vi "Configure Gamepad.vi"(4 "invert z":refnum<vi>, 6 "Cluster":T3, 7 "Configuration":T2, 8 "Slide 2":refnum<vi>, 9 "invert y":refnum<vi>, 10 "invert x":refnum<vi>, 11 "device ID":refnum<k1>) -> (3 "Configuration":T2)   [LabVIEW 2012]
uses:
  <vilib>/Utility/miscctls.llb/LVPointTypeDef.ctl
  <vilib>/Utility/inputDevices.llb/joystickAcquire.vi
  <vilib>/Utility/file.llb/Write To Spreadsheet File (I64).vi
  <vilib>/Utility/file.llb/Read From Spreadsheet File (I64).vi
panel:
  in  "Invert":bool=TRUE
  out "Settings Refrences":T1
  in  "M3+":u16(ring)=8 items=["1 X"=1, "2 A"=2, "3 B"=3, "4 Y"=4, "5 LB"=5, "6 RB"=6, "7 LT"=7, "8 RT"=8, "9 Back"=9]
  in  "M3-":u16(ring)=6 items=["1 X"=1, "2 A"=2, "3 B"=3, "4 Y"=4, "5 LB"=5, "6 RB"=6, "7 LT"=7, "8 RT"=8, "9 Back"=9]
  out "down":u16(ring) items=["M1+", "M1-", "M2+", "M2-"]
  out "left":u16(ring) items=["M1+", "M1-", "M2+", "M2-"]
  in  "right":u16(ring) items=["M1+", "M1-", "M2+", "M2-"]
  out "V":i32
  out "U":i32
  out "Left Y":i32
  out "B":i32
  out "A":i32
  out "Left X":i32
  out "Right Y":i32
  out "Right X":i32
  in  "close_button":bool
  in  "up":u16(ring) items=["M1+", "M1-", "M2+", "M2-"]
  in  "load":bool
  in  "save":bool
  in  "Invert":bool
  in  "Invert":bool=TRUE
  in  "Slide":cluster{u32, u32, u32}(slide)={7, 6, 2} scale=0.0..7.0
  in  "xr":u16(ring)=1 items=["1 X"=1, "2 A"=2, "3 B"=3, "4 Y"=4, "5 LB"=5, "6 RB"=6, "7 LT"=7, "8 RT"=8, "9 Back"=9]
  in  "yf":u16(ring)=4 items=["1 X"=1, "2 A"=2, "3 B"=3, "4 Y"=4, "5 LB"=5, "6 RB"=6, "7 LT"=7, "8 RT"=8, "9 Back"=9]
  in  "yr":u16(ring)=2 items=["1 X"=1, "2 A"=2, "3 B"=3, "4 Y"=4, "5 LB"=5, "6 RB"=6, "7 LT"=7, "8 RT"=8, "9 Back"=9]
  in  "xf":u16(ring)=3 items=["1 X"=1, "2 A"=2, "3 B"=3, "4 Y"=4, "5 LB"=5, "6 RB"=6, "7 LT"=7, "8 RT"=8, "9 Back"=9]
  in  "halt 2":u16(ring)=9 items=["1 X"=1, "2 A"=2, "3 B"=3, "4 Y"=4, "5 LB"=5, "6 RB"=6, "7 LT"=7, "8 RT"=8, "9 Back"=9]
  # "Control-sticks"
  # "Button mapping"
  # "Instructions\nDrag the M1 (green), M2 (red), and M3 (Blue)  MicroDrive-axis selectors to the name of a Gamepad Control-stick. \nNOTE: To identify your desired Control-stick, toggle the Control-stick while watching \"Readings\".\n\n."
  # "Instructions:\nClick on the text in a square to list Gamepad button options. The selected button will move the corresponding axis of the MicroDrive.\n\nThese settings effect the Gamepad buttons, and the  buttons/limit-lights of the main window."
  # "Axis"
  # "Selection"
  # "Readings"
  # "M1 Axis"
  # "M2 Axis"
  # "M3 Axis"
  # "CAUTION: The Gamepad's \"Mode\" button will disable the Control-sticks"
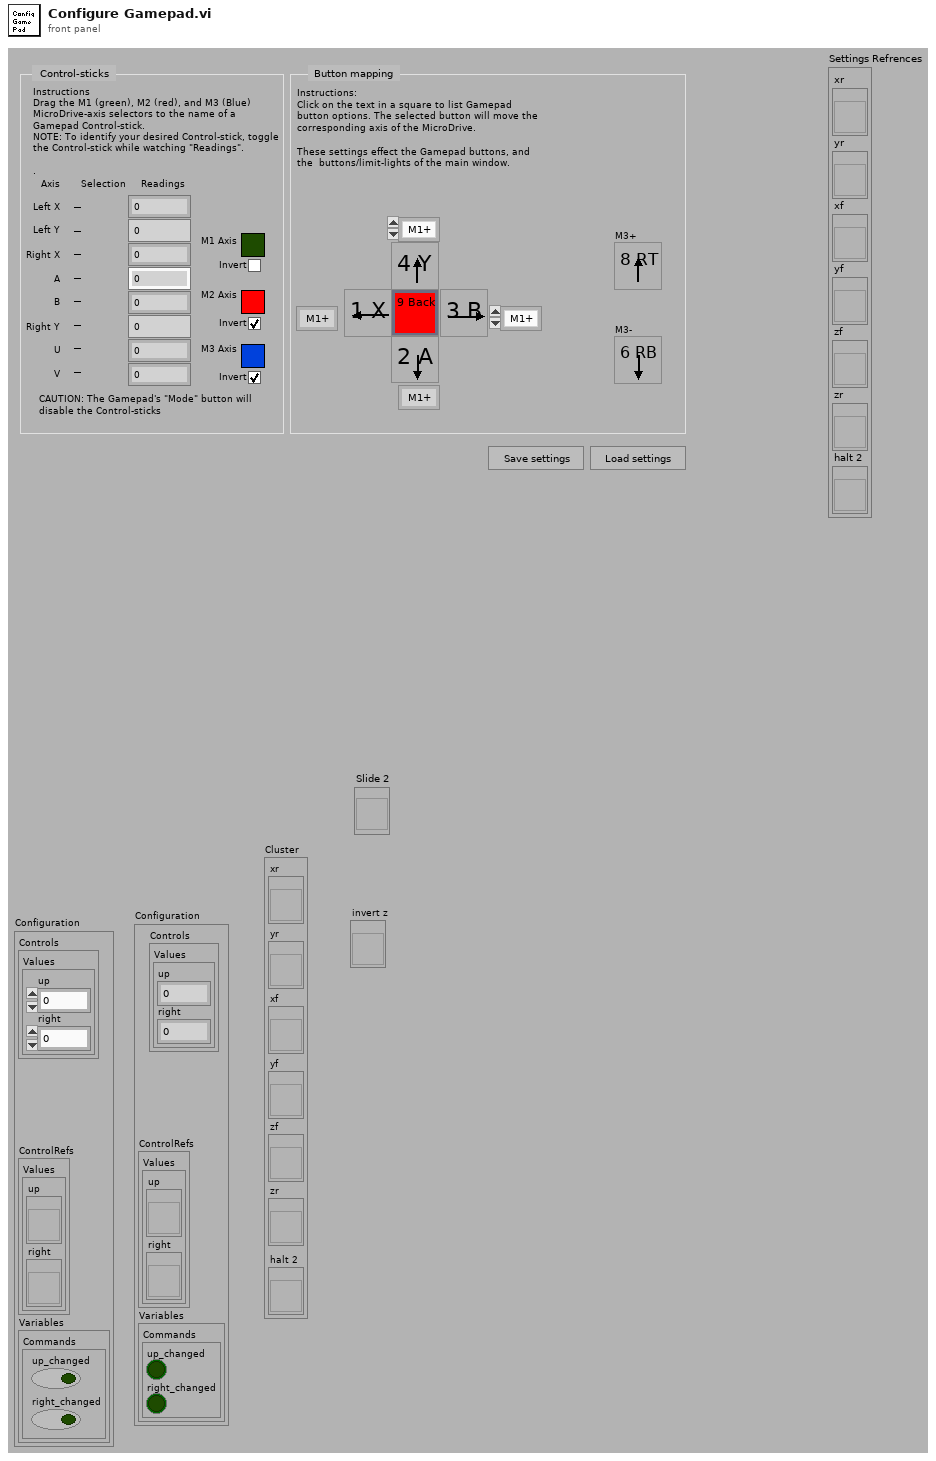
[diagram p1: front panel]
types:
  T1 = cluster{"xr":refnum<vi>, "yr":refnum<vi>, "xf":refnum<vi>, "yf":refnum<vi>, "zf":refnum<vi>, "zr":refnum<vi>, "halt 2":refnum<vi>}
  T2 = cluster{"Controls":cluster{"Values":cluster{"up":u16, "right":u16}}, "ControlRefs":cluster{"Values":cluster{"up":refnum<vi>, "right":refnum<vi>}}, "Variables":cluster{"Commands":cluster{"up_changed":bool, "right_changed":bool}}}
  T3 = cluster{"xr":refnum<vi>, "yr":refnum<vi>, "xf":refnum<vi>, "yf":refnum<vi>, "zr":refnum<vi>, "zf":refnum<vi>, "halt 2":refnum<vi>}
  T4 = typedef "LVPointTypeDef.ctl" = cluster{"Horizontal":i16, "Vertical":i16}
  T5 = cluster{"xr":refnum<vi>, "yr":refnum<vi>, "xf":refnum<vi>, "yf":refnum<vi>, "M3+":refnum<vi>, "M3-":refnum<vi>, "halt 2":refnum<vi>}
  T6 = cluster{"X axis":i32, "Y axis":i32, "Z axis":i32, "X axis rotation":i32, "Y axis rotation":i32, "Z axis rotation":i32, "U axis":i32, "V axis":i32}
  T7 = cluster{"Right X axis":i32, "Right Y axis":i32, "Left X axis":i32, "A Axis":i32, "B Axis":i32, "Left Y axis":i32, "U axis":i32, "V axis":i32}
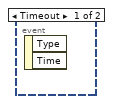
[diagram p2: hidden frame]
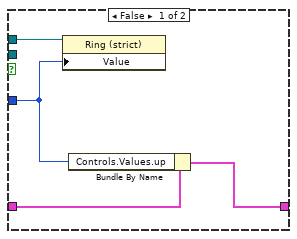
[diagram p4: hidden frame]
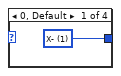
[diagram p5: hidden frame]
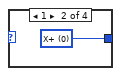
[diagram p6: hidden frame]
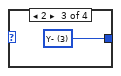
[diagram p7: hidden frame]
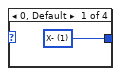
[diagram p8: hidden frame]
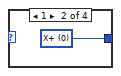
[diagram p9: hidden frame]
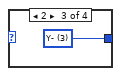
[diagram p10: hidden frame]
diagram:
  n1 = flat-sequence {
    tunnel: ["Configuration"] -> w9
    tunnel: w9 -> [w27]
    tunnel: [w26] -> w8
    tunnel: w8 -> [w29]
    tunnel: [w29] -> w22
    tunnel: [w28] -> w21
    tunnel: w22 -> [w31]
    tunnel: [w31] -> w20
    tunnel: w21 -> [w30]
    tunnel: [w35] -> w19
    tunnel: [w34] -> w18
    tunnel: w20 -> [w34]
    tunnel: [w44] -> w17
    tunnel: w19 -> [w44]
    tunnel: w18 -> [w43]
    tunnel: [w43] -> w16
    tunnel: w17 -> [w71]
    tunnel: [w71] -> w4
    tunnel: [w55] -> w2
    tunnel: w16 -> [w55]
    tunnel: w4 -> [w80]
    tunnel: [w80] -> w3
    tunnel: w2 -> [w79]
    tunnel: [w79] -> w1
    tunnel: [w82] -> w15
    tunnel: w3 -> [w82]
    tunnel: [w81] -> w14
    tunnel: w1 -> [w81]
    tunnel: w15 -> [w84]
    tunnel: [w84] -> w13
    tunnel: w14 -> [w83]
    tunnel: [w83] -> w12
    tunnel: w13 -> [w90]
    tunnel: w12 -> [w86]
    tunnel: [w88] -> w11
    tunnel: [w87] -> w10
    tunnel: w11 -> [w359]
    tunnel: w10 -> [w358]
    tunnel: [w359] -> w7
    tunnel: [w358] -> w5
    tunnel: w7 -> [w362]
    tunnel: [w362] -> w6
    tunnel: w5 -> [w361]
    tunnel: w6 -> [w363]
    frame #0 {
    }
    frame #1 {
      n2 = control-ref of="up"() -> (w25:refnum<vi>)
      n3 = control-ref of="right"() -> (w24:refnum<vi>)
      n4 = Bundle By Name(cluster=w27, "ControlRefs.Values.up"=w25, "ControlRefs.Values.right"=w24) -> (w26:T2)
    }
    frame #2 {
      n5 = control-ref of="This VI"() -> (w28:refnum<vi>)
    }
    frame #3 {
      w32 = FALSE ("Front Panel Window:Show Menu Bar")
      n6 = property class="VI"(reference=w30, "Front Panel.Minimizeable"=w32) -> ()  [unwired: 1 in, 2 out]
      n7 = property class="VI"(reference=w30, "Front Panel.ShowMenuBar"=w32) -> ()  [unwired: 1 in, 2 out]
      n8 = property class="VI"(reference=w30, "TB.Visible"=w32) -> ()  [unwired: 1 in, 2 out]
      n9 = property class="VI"(reference=w30, "Front Panel.Resizeable"=w32) -> ()  [unwired: 1 in, 2 out]
      n10 = property class="VI"(reference=w30, "Front Panel.Title"="Configure Gamepad" ("Front Panel Window:Title")) -> ()  [unwired: 1 in, 2 out]
    }
    frame #4 {
      n11 = control-ref of="This VI"() -> (w35:refnum<vi>)
      n12 = control-ref of="Pane"() -> (w36:refnum<vi>)
      n13 = property class="Pane"(reference=w36, "Origin"=T4 {"Horizontal"=0, "Vertical"=0}) -> ()  [unwired: 1 in, 2 out]
      n14 = property class="VI"(reference=w35, "GrowByDefault"=TRUE ("Expand When Dropped As SubVI")) -> ()  [unwired: 1 in, 2 out]
    }
    frame #5 {
      n15 = control-ref of="M3+"() -> (w39:refnum<vi>)
      n16 = control-ref of="halt 2"() -> (w42:refnum<vi>)
      n17 = control-ref of="M3-"() -> (w40:refnum<vi>)
      n18 = control-ref of="xr"() -> (w48:refnum<vi>)
      n19 = control-ref of="yr"() -> (w47:refnum<vi>)
      n20 = control-ref of="xf"() -> (w46:refnum<vi>)
      n21 = control-ref of="yf"() -> (w45:refnum<vi>)
      n22 = Bundle("xr"=w48, "yr"=w47, "xf"=w46, "yf"=w45, "M3+"=w39, "M3-"=w40, "halt 2"=w42) -> (→"Settings Refrences":T5)  [unwired: 1 out]
    }
    frame #6 {
      w50 = u32 7 ("x")
      n23 = local read "Settings Refrences"() -> (w54:T1)
      n24 = local read "Slide 2"() -> (w53:refnum<vi>)
      n25 = local read "Cluster"() -> (w58:T3)
      n26 = local read "invert x"() -> (w57:refnum<vi>)
      n27 = local read "invert y"() -> (w56:refnum<vi>)
      n28 = property on="Property Node" class="Slide (strict)"(reference=w53) -> ("Value"=w66:cluster{u32, u32, u32})  [unwired: 1 in, 2 out]
      n29 = Cluster To Array(cluster=w58) -> (array=w69:refnum<vi>[])
      n30 = Cluster To Array(cluster=w54) -> (array=w70:refnum<vi>[])
      n31 = property on="Property Node" class="Bool (strict)"(reference=w56) -> ("Value"=w62:bool)  [unwired: 1 in, 2 out]
      n32 = property on="Property Node" class="Bool (strict)"(reference=w57) -> ("Value"=w68:bool)  [unwired: 1 in, 2 out]
      n33 = for {
        tunnel: w70 -> [w73] mode=indexing
        tunnel: w69 -> [w74] mode=indexing
        n34 = property on="Property Node" class="Ring (strict)"(reference=w74) -> ("Value"=w72:u16)  [unwired: 1 in, 2 out]
        n35 = property on="Property Node" class="Ring (strict)"(reference=w73, "Value"=w72) -> ()  [unwired: 1 in, 2 out]
      }
      n36 = control-ref of="invert y"() -> (w59:refnum<vi>)
      n37 = Unbundle(w66) -> (w65:u32, w64:u32, w49:u32)
      n38 = control-ref of="invert x"() -> (w61:refnum<vi>)
      n39 = Subtract(x=w50, y=w65) -> (x-y=w52:u32)
      n40 = Subtract(x=w50, y=w64) -> (x-y=w63:u32)
      n41 = Subtract(x=w50, y=w49) -> (x-y=w51:u32)
      n42 = property on="Property Node" class="Bool (strict)"(reference=w59, "Value"=w62) -> ()  [unwired: 1 in, 2 out]
      n43 = property on="Property Node" class="Bool (strict)"(reference=w61, "Value"=w68) -> ()  [unwired: 1 in, 2 out]
      n44 = control-ref of="Slide"() -> (w60:refnum<vi>)
      n45 = Bundle(w52, w63, w51) -> (w67:cluster{u32, u32, u32})  [unwired: 1 out]
      n46 = property on="Property Node" class="Slide (strict)"(reference=w60, "Value"=w67) -> ()  [unwired: 1 in, 2 out]
    }
    frame #7 {
      n47 = Unbundle By Name(w79) -> ("ControlRefs.Values.up"=w78:refnum<vi>, "Controls.Values.up"=w77:u16, "ControlRefs.Values.right"=w76:refnum<vi>, "Controls.Values.right"=w75:u16)
      n48 = property class="Ring (strict)"(reference=w78, "Value"=w77) -> ()  [unwired: 1 in, 2 out]
      n49 = property class="Ring (strict)"(reference=w76, "Value"=w75) -> ()  [unwired: 1 in, 2 out]
    }
    frame #8 {
    }
    frame #9 {
      n50 = property class="VI"(reference=w84, "GrowByDefault"=FALSE ("Expand When Dropped As SubVI")) -> ()  [unwired: 1 in, 2 out]
    }
    frame #10 {
      n51 = while {
        tunnel: w90 -> [w136]
        tunnel: [w99] -> w88
        shift-right: [w98] -> w87
        shift-left: w86 -> [w97]
        stop <- w135 stop-if-true
        n52 = flat-sequence {
          tunnel: w136 -> [w137]
          tunnel: w97 -> [w138]
          tunnel: [w138] -> w121
          tunnel: [w137] -> w109
          tunnel: [w148] -> w112
          tunnel: w121 -> [w147]
          tunnel: [w140] -> w110
          tunnel: w109 -> [w140]
          tunnel: w112 -> [w150]
          tunnel: [w149] -> w111
          tunnel: w110 -> [w151]
          tunnel: [w151] -> w108
          tunnel: [w189] -> w120
          tunnel: w111 -> [w189]
          tunnel: w108 -> [w188]
          tunnel: [w188] -> w106
          tunnel: ["Slide"] -> w126
          tunnel: [w211] -> w124
          tunnel: [w210] -> w122
          tunnel: w120 -> [w209]
          tunnel: [w209] -> w118
          tunnel: [w208] -> w107
          tunnel: w106 -> [w208]
          tunnel: w126 -> [w235]
          tunnel: [w235] -> w125
          tunnel: w124 -> [w234]
          tunnel: [w234] -> w123
          tunnel: w122 -> [w233]
          tunnel: [w224] -> w119
          tunnel: w118 -> [w224]
          tunnel: w107 -> [w223]
          tunnel: [w223] -> w104
          tunnel: [w244] -> w134
          tunnel: [w243] -> w133
          tunnel: w125 -> [w243]
          tunnel: [w242] -> w130
          tunnel: w123 -> [w241]
          tunnel: [w241] -> w127
          tunnel: w119 -> [w240]
          tunnel: [w240] -> w117
          tunnel: [w239] -> w105
          tunnel: w104 -> [w239]
          tunnel: w134 -> [w259]
          tunnel: w133 -> [w258]
          tunnel: [w258] -> w132
          tunnel: w130 -> [w260]
          tunnel: [w260] -> w128
          tunnel: w127 -> [w249]
          tunnel: w117 -> [w252]
          tunnel: [w252] -> w116
          tunnel: w105 -> [w253]
          tunnel: [w253] -> w103
          tunnel: w132 -> [w294]
          tunnel: [w294] -> w131
          tunnel: [w292] -> w129
          tunnel: w128 -> [w292]
          tunnel: w116 -> [w289]
          tunnel: [w289] -> w114
          tunnel: w103 -> [w290]
          tunnel: [w290] -> w102
          tunnel: w131 -> [_]
          tunnel: w129 -> [_]
          tunnel: [w328] -> w115
          tunnel: w114 -> [w328]
          tunnel: w102 -> [w327]
          tunnel: [w327] -> w100
          tunnel: w115 -> [w337]
          tunnel: [w337] -> w113
          tunnel: [w336] -> w101
          tunnel: w100 -> [w336]
          tunnel: [w346] -> w96
          tunnel: w113 -> [w346]
          tunnel: [w345] -> w94
          tunnel: w101 -> [w345]
          tunnel: w96 -> [w354]
          tunnel: [w354] -> w95
          tunnel: w94 -> [w353]
          tunnel: [w353] -> w93
          tunnel: ["close_button"] -> w135
          tunnel: w95 -> [w356]
          tunnel: [w356] -> w98
          tunnel: w93 -> [w355]
          tunnel: [w355] -> w99
          frame #0 {
            n53 = property class="VI"(reference=w137, "Front Panel.IsFrontmost"=TRUE ("Front Panel Window:Is Frontmost")) -> ()  [unwired: 1 in, 2 out]
          }
          frame #1 {
            n54 = Unbundle By Name(w147) -> ("Controls.Values.up"=w144:u16, "Controls.Values.right"=w145:u16)
            n55 = Not Equal?(x="up", y=w144) -> (x != y?=w146:bool)
            n56 = Not Equal?(x=w145, y="right") -> (x != y?=w141:bool)
            n57 = Bundle By Name(cluster=w147, "Controls.Values.up"="up", "Controls.Values.right"="right", "Variables.Commands.up_changed"=w146, "Variables.Commands.right_changed"=w141) -> (w148:T2)
          }
          frame #2 {
            n58 = Unbundle By Name(w150) -> ("Controls.Values.up"=w169:u16, "Controls.Values.right"=w166:u16)
            n59 = Unbundle By Name(w150) -> ("Controls.Values.up"=w158:u16, "Controls.Values.right"=w161:u16)
            n60 = Unbundle By Name(w150) -> ("ControlRefs.Values.up"=w154:refnum<vi>, "ControlRefs.Values.right"=w153:refnum<vi>, "Variables.Commands.up_changed"=w155:bool)
            n61 = Less Or Equal?(x=w166, y=u16 1) -> (x <= y?=w164:bool)
            n62 = Greater?(x=w161, y=u16 1) -> (0:w163:bool)
            n63 = Less Or Equal?(x=w169, y=u16 1) -> (x <= y?=w165:bool)
            n64 = Greater?(x=w158, y=u16 1) -> (0:w162:bool)
            n65 = Compound Arithmetic op=AND(w165, w164) -> (w152:bool)
            n66 = Compound Arithmetic op=AND(w162, w163) -> (w157:bool)
            n67 = Compound Arithmetic op=OR(w152, w157) -> (w156:bool)
            n68 = case shown="True" w156 {
              tunnel: w155 -> [_ w179]
              tunnel: w154 -> [_ w178]
              tunnel: w153 -> [_ w177]
              tunnel: w152 -> [_ w176]
              tunnel: w150 -> [w170 w172]
              tunnel: [w170 w171] -> w149
              frame False {
              }
              frame True {
                n69 = Select(t=u16 2 ("Controls.Values.up"), s=w176, f=u16 1 ("Controls.Values.up")) -> (s? t:f=w173:u16)
                n70 = case shown="True" w179 {
                  tunnel: w178 -> [w183 _]
                  tunnel: w177 -> [_ w187]
                  tunnel: w173 -> [w180 w184]
                  tunnel: w172 -> [w182 w186]
                  tunnel: [w181 w185] -> w171
                  frame False {
                    n71 = property class="Ring (strict)"(reference=w183, "Value"=w180) -> ()  [unwired: 1 in, 2 out]
                    n72 = Bundle By Name(cluster=w182, "Controls.Values.up"=w180) -> (w181:T2)
                  }
                  frame True {
                    n73 = Bundle By Name(cluster=w186, "Controls.Values.right"=w184) -> (w185:T2)
                    n74 = property class="Ring (strict)"(reference=w187, "Value"=w184) -> ()  [unwired: 1 in, 2 out]
                  }
                }
              }
            }
          }
          frame #3 {
            n75 = Unbundle By Name(w189) -> ("Controls.Values.right"=w191:u16)
            n76 = Unbundle By Name(w189) -> ("Controls.Values.up"=w190:u16)
            n77 = case shown="3" w190 {
              tunnel: [w198 w199 w200 w201] -> w193
              frame 0, Default {
                w198 = u16 1 items=["X+", "X-", "Y+", "Y-"] ("up")
              }
              frame 1 {
                w199 = u16 0 items=["X+", "X-", "Y+", "Y-"] ("up")
              }
              frame 2 {
                w200 = u16 3 items=["X+", "X-", "Y+", "Y-"] ("up")
              }
              frame 3 {
                w201 = u16 2 items=["X+", "X-", "Y+", "Y-"] ("up")
              }
            }
            "down" <- w193
            n78 = case shown="3" w191 {
              tunnel: [w194 w195 w196 w197] -> w192
              frame 0, Default {
                w194 = u16 1 items=["X+", "X-", "Y+", "Y-"] ("up")
              }
              frame 1 {
                w195 = u16 0 items=["X+", "X-", "Y+", "Y-"] ("up")
              }
              frame 2 {
                w196 = u16 3 items=["X+", "X-", "Y+", "Y-"] ("up")
              }
              frame 3 {
                w197 = u16 2 items=["X+", "X-", "Y+", "Y-"] ("up")
              }
            }
            "left" <- w192
          }
          frame #4 {
            w203 = u32 7 ("x")
            n79 = Unbundle("Slide") -> (w218:u32, w219:u32, w202:u32)
            n80 = Subtract(x=w203, y=w218) -> (x-y=w220:u32)
            n81 = Subtract(x=w203, y=w202) -> (x-y=w205:u32)
            n82 = Subtract(x=w203, y=w219) -> (x-y=w221:u32)
            n83 = call-poly <vilib>:"Acquire Input Data.vi"("device ID"="device ID") -> ("axis info"=w216:T6)  [unwired: 1 in, 17 out]
            n84 = Bundle(cluster="Slide", w220, w221, w205) -> (w222:cluster{u32, u32, u32})
            n85 = call "invert joystick cluster values.vi"("Invert Z"="Invert", "Invert Y"="Invert", "Invert X"="Invert", "Slide"=w222, "Joystick Readings"=w216) -> ("Joystick Readings 2"=w210:T7)  [unwired: 6 out]
            n86 = Boolean To (0,1)(Boolean="Invert") -> (0, 1=w213:i16)
            n87 = Boolean To (0,1)(Boolean="Invert") -> (0, 1=w212:i16)
            n88 = Boolean To (0,1)(Boolean="Invert") -> (0, 1=w207:i16)
            n89 = Build Array(w213, w212, w207) -> (w211:i16[])
          }
          frame #5 {
            n90 = Unbundle By Name(w233) -> ("Right X axis"=→"Left X":i32, "Right Y axis"=→"Left Y":i32, "Left X axis"=→"Right X":i32, "A Axis"=→"A":i32, "B Axis"=→"B":i32, "Left Y axis"=→"Right Y":i32, "U axis"=→"U":i32, "V axis"=→"V":i32)
          }
          frame #6 {
            n91 = local read "Settings Refrences"() -> (w238:T1)
            n92 = Cluster To Array(cluster="Cluster") -> (array=w236:refnum<vi>[])
            n93 = Cluster To Array(cluster=w238) -> (array=w242:refnum<vi>[])
            n94 = for {
              tunnel: w242 -> [w247] mode=indexing
              tunnel: [w245] -> w244 mode=indexing
              tunnel: w236 -> [w246] mode=indexing
              n95 = property on="Property Node" class="Ring (strict)"(reference=w247) -> ("Value"=w245:u16)  [unwired: 1 in, 2 out]
              n96 = property on="Property Node" class="Ring (strict)"(reference=w246, "Value"=w245) -> ()  [unwired: 1 in, 2 out]
            }
          }
          frame #7 {
            n97 = Unbundle By Name(w252) -> ("Controls.Values.up"=w250:u16, "Controls.Values.right"=w251:u16)
            n98 = Unbundle(w258) -> (w257:u32, w256:u32, w248:u32)
            n99 = Build Array (concatenate)(w259, w257, w256, w248, w249, w250, w251) -> (w255:u32[])
            n100 = case shown="True" "save" {
              tunnel: w255 -> [_ w276]
              frame False {
              }
              frame True {
                n101 = Get Date/Time String() -> (date string=w264:string, time string=w273:string)  [unwired: 3 out]
                n102 = call <vilib>:"Space Constant.vi"() -> ("String"=w272:string)
                n103 = Concatenate Strings(w264, w272, w273) -> (w265:string)
                n104 = control-ref of="This Application"() -> (w280:refnum<vi>)
                n105 = Search and Replace String(replace all?=TRUE ("replace all? (F)"), input string=w265, search string=":") -> (result string=w267:string)  [unwired: 1 in, 7 out]
                n106 = Search and Replace String(replace all?=TRUE ("replace all? (F)"), input string=w267, search string="/", replace string="-" ("replace string (\"\")")) -> (result string=w263:string)  [unwired: 1 in, 6 out]
                n107 = property class="App"(reference=w280) -> ("App.Dir"=w282:path)  [unwired: 1 in, 2 out]
                n108 = Concatenate Strings("gamepad  " ("string"), w263) -> (w261:string)
                n109 = call "File Dialog"("default name"=w261, "pattern (all files)"="*.txt") -> ("selected path"=w278:path, "cancelled"=w277:bool, "error out"=w274:errorcluster)  [unwired: 5 in, 6 out]
                n110 = Build Path(base path=w282, name or relative path="config.txt") -> (appended path=w279:path)
                n111 = case shown="False" w277 {
                  tunnel: w279 -> [w288 _]
                  tunnel: w278 -> [w284 _]
                  tunnel: w276 -> [w283 _]
                  tunnel: w274 -> [_ _]
                  frame False {
                    n112 = call-poly <vilib>:"Write To Spreadsheet File.vi"("transpose? (no:F)"=TRUE, "1D data"=w283, "file path (dialog if empty)"=w284) -> ("new file path (Not A Path if cancelled)"=w287:path)  [unwired: 3 in, 2 out]
                    n113 = Path To String(path=w287) -> (string=w285:string)
                    n114 = Write to Text File(file (use dialog)=w288, text=w285) -> ()  [unwired: 1 in, 4 out]
                  }
                  frame True {
                  }
                }
              }
            }
          }
          frame #8 {
            n115 = control-ref of="Slide"() -> (w291:refnum<vi>)
            n116 = case shown="True" "load" {
              tunnel: w292 -> [_ w300]
              tunnel: w291 -> [_ w301]
              tunnel: w289 -> [_ w295]
              frame False {
              }
              frame True {
                n117 = call "File Dialog2"("pattern (all files)"="*.txt") -> ("selected path"=w298:path, "cancelled"=w296:bool, "error out"=w297:errorcluster)  [unwired: 6 in, 6 out]
                n118 = case shown="False" w296 {
                  tunnel: w301 -> [w307 _]
                  tunnel: w300 -> [w319 _]
                  tunnel: w298 -> [w311 _]
                  tunnel: w297 -> [_ _]
                  tunnel: w295 -> [w308 _]
                  frame False {
                    n119 = call-poly <vilib>:"Read From Spreadsheet File.vi"("transpose (no:F)"=TRUE ("transpose? (no:F)"), "file path (dialog if empty)"=w311) -> ("first row"=w312:i64[])  [unwired: 2 in, 7 out]
                    n120 = Array Size(array=w319) -> (size(s)=w324:i32)
                    n121 = Split 1D Array(array=w312, index=w324) -> (first subarray=w318:i64[], second subarray=w323:i64[])
                    n122 = Index Array(array=w323) -> (element #1=w321:i64, element #2=w322:i64, element #3=w302:i64, element #4=w303:i64, element #5=w304:i64, element #6=w305:i64, element #7=w306:i64)  [unwired: 7 in]
                    n123 = Bundle(w321, w322, w302) -> (w320:cluster{i64, i64, i64})  [unwired: 1 out]
                    n124 = property class="Slide (strict)"(reference=w307, "Value"=w320) -> ()  [unwired: 1 in, 2 out]
                    n125 = control-ref of="Invert"() -> (w317:refnum<vi>)
                    n126 = Greater Than 0?(x=w303) -> (x > 0?=w315:bool)
                    n127 = property class="Bool (strict)"(reference=w317, "Value"=w315) -> ()  [unwired: 1 in, 2 out]
                    n128 = control-ref of="Invert"() -> (w316:refnum<vi>)
                    n129 = Greater Than 0?(x=w304) -> (x > 0?=w314:bool)
                    n130 = property class="Bool (strict)"(reference=w316, "Value"=w314) -> ()  [unwired: 1 in, 2 out]
                    n131 = Unbundle By Name(w308) -> ("ControlRefs.Values.up"=w310:refnum<vi>)
                    n132 = property class="Ring (strict)"(reference=w310, "Value"=w305) -> ()  [unwired: 1 in, 2 out]
                    n133 = Unbundle By Name(w308) -> ("ControlRefs.Values.right"=w309:refnum<vi>)
                    n134 = property class="Ring (strict)"(reference=w309, "Value"=w306) -> ()  [unwired: 1 in, 2 out]
                    n135 = for {
                      tunnel: w319 -> [w326] mode=indexing
                      tunnel: w318 -> [w325] mode=indexing
                      n136 = property class="Ring (strict)"(reference=w326, "Value"=w325) -> ()  [unwired: 1 in, 2 out]
                    }
                  }
                  frame True {
                  }
                }
              }
            }
          }
          frame #9 {
            n137 = control-ref of="invert x"() -> (w330:refnum<vi>)
            n138 = property on="Property Node" class="Bool (strict)"(reference=w330) -> ("Value"=w329:bool)  [unwired: 1 in, 2 out]
            n139 = property on="Property Node" class="Bool (strict)"(reference="invert x", "Value"=w329) -> ()  [unwired: 1 in, 2 out]
          }
          frame #10 {
            w333 = u32 7 ("x")
            n140 = control-ref of="Slide"() -> (w338:refnum<vi>)
            n141 = property on="Property Node" class="Slide (strict)"(reference=w338) -> ("Value"=w343:cluster{u32, u32, u32})  [unwired: 1 in, 2 out]
            n142 = Unbundle(w343) -> (w342:u32, w341:u32, w332:u32)
            n143 = Subtract(x=w333, y=w342) -> (x-y=w340:u32)
            n144 = Subtract(x=w333, y=w341) -> (x-y=w339:u32)
            n145 = Subtract(x=w333, y=w332) -> (x-y=w334:u32)
            n146 = Bundle(w340, w339, w334) -> (w344:cluster{u32, u32, u32})  [unwired: 1 out]
            n147 = property on="Property Node" class="Slide (strict)"(reference="Slide 2", "Value"=w344) -> ()  [unwired: 1 in, 2 out]
          }
          frame #11 {
            n148 = control-ref of="invert y"() -> (w348:refnum<vi>)
            n149 = property on="Property Node" class="Bool (strict)"(reference=w348) -> ("Value"=w347:bool)  [unwired: 1 in, 2 out]
            n150 = property on="Property Node" class="Bool (strict)"(reference="invert y", "Value"=w347) -> ()  [unwired: 1 in, 2 out]
          }
          frame #12 {
            n151 = control-ref of="Invert"() -> (w350:refnum<vi>)
            n152 = property on="Property Node" class="Bool (strict)"(reference=w350) -> ("Value"=w351:bool)  [unwired: 1 in, 2 out]
            n153 = property on="Property Node" class="Bool (strict)"(reference="invert z", "Value"=w351) -> ()  [unwired: 1 in, 2 out]
          }
          frame #13 {
          }
        }
      }
      n154 = event shown="[1] Panel Close?" {
        selector: _ -> [_ _]
        dyn-events: _ -> [_ _]
        timeout: -1 -> [_ _]
        event Timeout {
          n155 = event-data() -> ()  [unwired: 3 out]
        }
        event Panel Close? {
          n156 = event-data() -> ()  [unwired: 4 out]
          n157 = local write "close_button"(TRUE ("closed?")) -> ()
          n158 = event-data("Discard?"=TRUE) -> ()  [unwired: 1 in, 1 out]
        }
      }
    }
    frame #11 {
      w360 = FALSE  # close_button
      n159 = local write "close_button"(w360) -> ()
    }
    frame #12 {
      "Configuration" <- w361
    }
    frame #13 {
      n160 = invoke class="VI" method="FP.Close"(reference=w363) -> ()  [unwired: 2 in, 3 out]
    }
  }
